vi "Open Transport Server.vi"(8 "error in (no error)":errorcluster) -> (0 "error out":errorcluster)   [LabVIEW 2019, in "Control Experiment.lvclass"]
uses:
  Control Experiment.lvclass
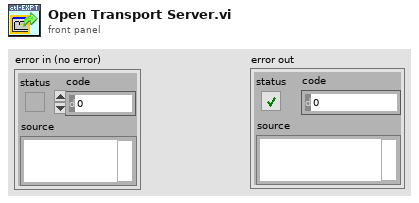
[diagram p1: front panel]
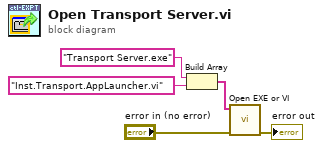
[diagram p0: block diagram]
diagram:
  n1 = Build Array("Transport Server.exe" ("pattern"), "Inst.Transport.AppLauncher.vi" ("pattern")) -> (w1:string[])
  n2 = call "Open EXE or VI.vi"("error in (no error)"="error in (no error)", "Paths"=w1) -> ("error out"=→"error out":errorcluster)  [unwired: 9 in]
